vi "read_params.vi"(8 "error in (no error)":errorcluster, 11 "MultiTaskLassoCV in":refnum<class "MultiTaskLassoCV.lvclass">) -> (0 "error out":errorcluster, 2 "params":T1={"eps"=0.001, "n_alphas"=100.0, "alphas"={"alphas_type"="None", "alphas_list"=[]}, "fit_intercept"=TRUE, "normalize"=FALSE, "max_iter"=1000.0, "tol"=0.0001, "copy_X"=TRUE, "cv"=5.0, "verbose"={"verbose_type"="bool", "verbose_int"=0.0, "verbose_bool"=FALSE}, "n_jobs"=1.0, "random_state"=0.0, "selection"="cyclic"}, 3 "MultiTaskLassoCV out":refnum<class "MultiTaskLassoCV.lvclass">)   [LabVIEW 2020, in "MultiTaskLassoCV.lvclass"]
uses:
  MultiTaskLassoCV.lvclass
  Controls/multi_task_lasso_cv_params.ctl
  MultiTaskLassoCV.lvclass/MultiTaskLassoCV.ctl
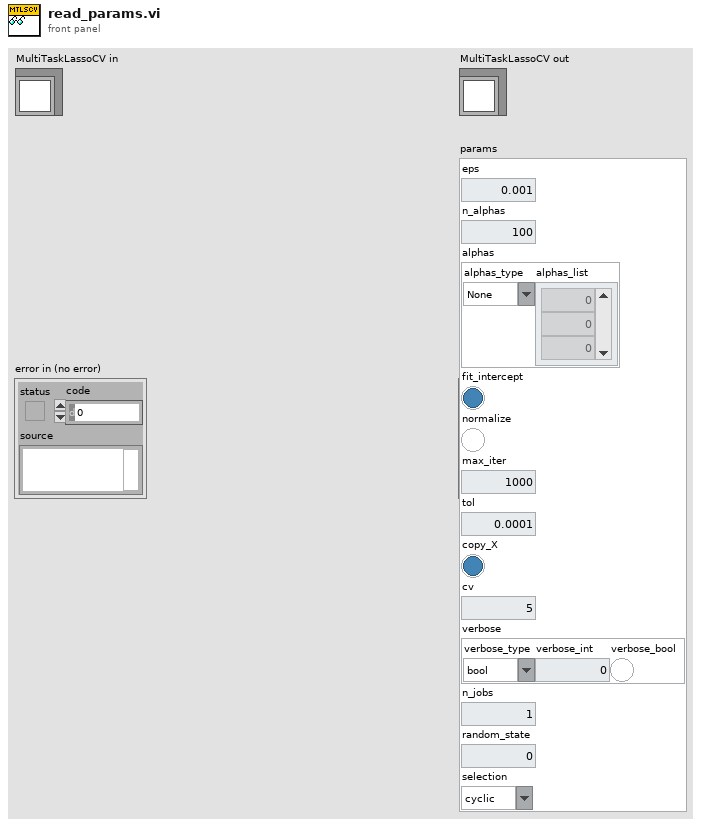
[diagram p1: front panel]
types:
  T1 = typedef "multi_task_lasso_cv_params.ctl" = cluster{"eps":dbl, "n_alphas":dbl, "alphas":cluster{"alphas_type":string, "alphas_list":dbl[]}, "fit_intercept":bool, "normalize":bool, "max_iter":dbl, "tol":dbl, "copy_X":bool, "cv":dbl, "verbose":cluster{"verbose_type":string, "verbose_int":dbl, "verbose_bool":bool}, "n_jobs":dbl, "random_state":dbl, "selection":string}
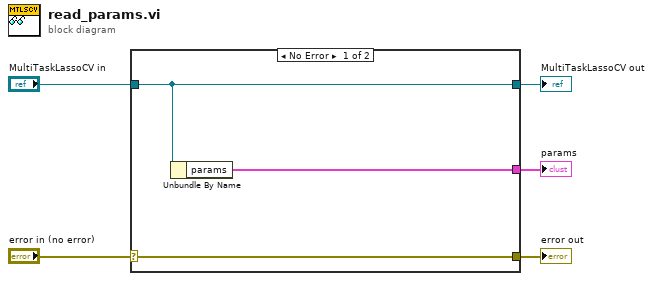
[diagram p0: block diagram]
diagram:
  n1 = case shown="No Error" "error in (no error)" {
    selector: "error in (no error)" -> [w8 w9]
    tunnel: [w8 w9] -> w4
    tunnel: [w7 w10] -> w2
    tunnel: "MultiTaskLassoCV in" -> [w7 w10]
    tunnel: [w6 _] -> w1
    frame No Error {
      n2 = Unbundle By Name(w7) -> ("params"=w6:T1)
    }
    frame Error {
    }
  }
  "error out" <- w4
  "MultiTaskLassoCV out" <- w2
  "params" <- w1
